vi "ConnectToSQL.vi"() -> (0 "error out":errorcluster, 1 "connection reference":T1)   [LabVIEW 2023]
uses:
  <vilib>/addons/database/Connection.llb/DB Tools Open Connec (Path).vi
  <vilib>/addons/database/NI_Database_API.lvlib
  <vilib>/addons/database/Connection.llb/Conn ObjectReference.ctl
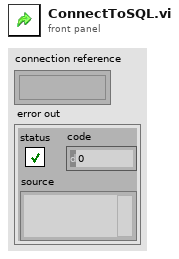
[diagram p1: front panel]
types:
  T1 = typedef "NI_Database_API.lvlib/Conn ObjectReference.ctl" = refnum<k1>
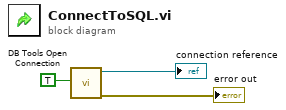
[diagram p0: block diagram]
diagram:
  n1 = call-poly <vilib>:"DB Tools Open Connection.vi"("prompt? (F)"=TRUE) -> ("error out"=→"error out":errorcluster, "connection reference"=→"connection reference":T1)  [unwired: 7 in]
